vi "Measuring average over input data.vi"() -> ()   [LabVIEW 2020]
uses:
  <vilib>/Analysis/baseanly.llb/Mean (DBL).vi
  <vilib>/Analysis/NI_AALBase.lvlib
panel:
  out "path":path=path "C:/Users/htm22/Documents/LabVIEW Data/test_020.lvm"
  out "Average values over samples":dbl[](graph)=[-0.06588994800000003, -0.053160485000000146, -0.04160002399999998, -0.03074547999999998, -0.020515026000000013, -0.010707168788300029, -0.0012061949999999926, 0.007962175642339996, 0.016884849927020003, 0.025614471642340018, 0.03410596699999997, 0.04241317099999998, 0.050556878999999916, 0.05854111000000014, 0.06634789399999985, 0.07399698800000008, 0.08149821199999989, 0.08882978599999994, 0.09602468900000025, 0.10301141099999984]
  out "Incoming data":dynamicdata(graph)=[{"t0"=timestamp(0 s since 1904-01-01), "dt"=1.0, "Y"=array[1000 elements], "attributes"=variant("NI_ChannelName"=variant(string "Untitled"), "NI_ExpIsRelativeTime"=variant(bool TRUE), "NI_ExpStartTimeStamp"=variant(timestamp timestamp(3780594175.2018385 s since 1904-01-01)), "NI_ExpTimeStamp"=variant(timestamp timestamp(0 s since 1904-01-01)), "NI_ExpXDimension"=variant(string "t"), "NI_UnitDescription"=variant(string "V"))}]
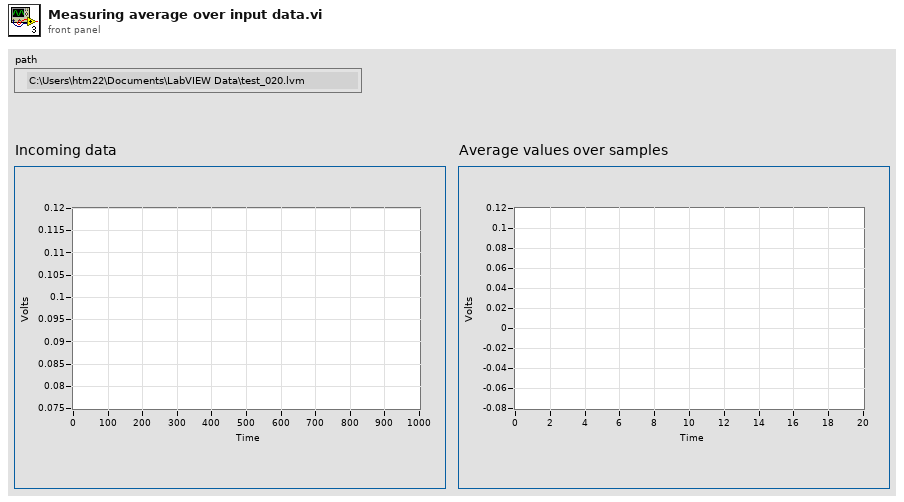
[diagram p1: front panel]
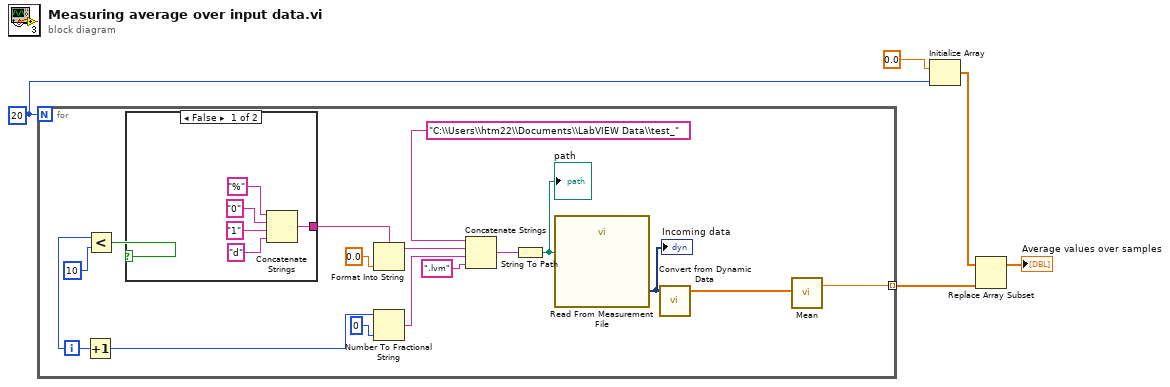
[diagram p0: block diagram]
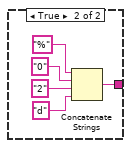
[diagram p2: hidden frame]
diagram:
  w1 = 20
  n1 = for {
    N: w1 -> [_]
    tunnel: [w20] -> w3 mode=indexing
    i -> [w11]
    n2 = Increment(x=w11) -> (x+1=w10:i32)
    n3 = Less?(x=w10, y=10) -> (x < y?=w8:bool)
    n4 = case shown="False" w8 {
      tunnel: [w22 w27] -> w7
      frame False {
        n5 = Concatenate Strings("%" ("string"), "0" ("string"), "1" ("string"), "d" ("string")) -> (w22:string)
      }
      frame True {
        n6 = Concatenate Strings("%" ("string"), "0" ("string"), "2" ("string"), "d" ("string")) -> (w27:string)
      }
    }
    n7 = Format Into String(format string=w7, 0.0 ("input 1")) -> (resulting string=w12:string)  [unwired: 2 in, 1 out]
    n8 = Number To Fractional String(number=w10, precision (6)=i16 0) -> (F-format string=w13:string)  [unwired: 2 in]
    n9 = Concatenate Strings("C:\\Users\\htm22\\Documents\\LabVIEW Data\\test_" ("string"), w12, w13, ".lvm") -> (w18:string)
    n10 = String To Path(string=w18) -> (path=w19:path)
    "path" <- w19
    n11 = call "Read From Measurement File"("Filename"=w19) -> ("Signals"=w21:dynamicdata)  [unwired: 5 in, 5 out]
    "Incoming data" <- w21
    n12 = call "Convert from Dynamic Data"("Dynamic Data Type"=w21) -> ("Array"=w6:dbl[])  [unwired: 3 in]
    n13 = call-poly <vilib>:"Mean.vi"("X"=w6) -> ("mean"=w20:dbl)  [unwired: 1 out]
  }
  n14 = Initialize Array(0.0 ("element"), w1) -> (w4:dbl[])
  n15 = Replace Array Subset(array=w4, new element=w3) -> (→"Average values over samples":dbl[])  [unwired: 1 in]
